vi "Program Deinitialization.vi"(8 "error in":errorcluster, 11 "classes in":T1) -> (0 "error out":errorcluster, 3 "classes out":T1)   [LabVIEW 2011]
uses:
  Controls/Class Objects.ctl
  Modules/File/Configuration/Configuration.lvclass
  Modules/Hardware/Power Supply/Power Supply.lvclass
  Modules/Hardware/Mass Flow Controller/Mass Flow Controller.lvclass
  Modules/Hardware/PID/PID.lvclass
  Modules/Hardware/Valve Controller/Valve Controller.lvclass
  Modules/Hardware/Multimeter/Multimeter.lvclass
  Modules/Hardware/Vapour Generator/Vapour Generator.lvclass
  Modules/File/TDMS/TDMS.lvclass
  Controls/Class Labels.ctl
  Functional Global Data/Globals.ctl
  Functional Global Data/Device Params Global.ctl
  Controls/User Interface Action.ctl
  Controls/Display Mode.ctl
  Functional Global Data/Analysis Data.ctl
  Functional Global Data/Run Data.ctl
  Modules/Menu/Menu Action.ctl
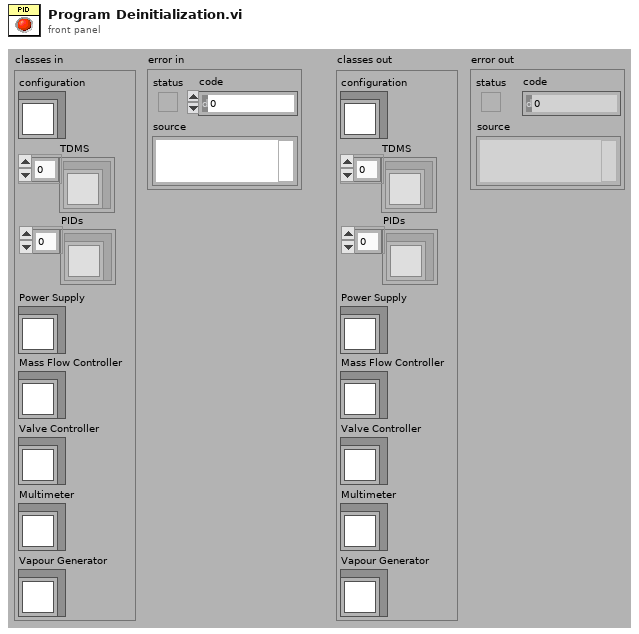
[diagram p1: front panel]
types:
  T1 = typedef "Class Objects.ctl" = cluster{"configuration":refnum<class "Configuration.lvclass">, "TDMS":refnum<class "TDMS.lvclass">[], "Power Supply":refnum<class "Power Supply.lvclass">, "Mass Flow Controller":refnum<class "Mass Flow Controller.lvclass">, "Valve Controller":refnum<class "Valve Controller.lvclass">, "Multimeter":refnum<class "Multimeter.lvclass">, "Vapour Generator":refnum<class "Vapour Generator.lvclass">, "PIDs":refnum<class "PID.lvclass">[]}
  T2 = typedef "Class Labels.ctl" = enum16{"Configuration", "TDMS", "PID", "Power Supply", "Vapour Generator", "MFC", "NMR", "Valve Controller", "Multimeter"}
  T3 = typedef "Globals.ctl" = enum16{"Initialize", "Get DAQ Params", "Get Data Display Params", "Set DAQ Params", "Set Data Display Params"}
  T4 = typedef "Device Params Global.ctl" = enum16{"Initialize", "Get Device Settings", "Get Device Connections", "Set Device Settings", "Set Device Connections", "Get All Device Properties"}
  T5 = typedef "User Interface Action.ctl" = enum16{"Initialize", "Data Acquisition Disable", "Data View Disable", "Sample Set", "Sample Set 2D Data", "Sample Set x0 & dx", "Sample Add", "Sample Set Cursor", "Sample Set Offset & Multiplier", "Sample Set Axis Labels", "Sample Parameters Disabled", "Sample Parameters Update", "Run Update", "Run Set Offset & Multiplier", "Run Set Axis Labels", "Run Set Cursor", "Run Set Disabled", "Run Parameters Update", "Run Parameters Disabled", "Run Number Set", "Run Number Set Range", "Run Number Set Disabled", "Sample Number Set", "Sample Number Set Range", "Notes Set Value", "Update Plot", "Set Plot Parameters", "Update Concentration Plot", "Time Set", "Clear DAQ Display", "Clear Analysis Display", "Status Bar Set", "Progress Bar Set", "Display Mode Set", "Experiment Type Set", "Analysis Plot Average Set", "Stop"}
  T6 = typedef "Display Mode.ctl" = enum16{"Sample", "Run"}
  T7 = typedef "Analysis Data.ctl" = enum16{"Initialize", "Add Plot", "Get Plots"}
  T8 = typedef "Run Data.ctl" = enum16{"Initialize", "Add Sample Channel", "Set Run", "Get Number of Runs", "Set Run Params", "Get Spectrum", "Get Run Params", "Get Sample Params", "Get History", "Get Averaged History", "Get Run Param Names", "Set Run Param Names", "Get Sample Param Names", "Set Sample Param Names", "Get MFC Flow Rate Challenge Profile", "Get History Average"}
  T9 = typedef "Menu Action.ctl" = enum16{"Initialize", "Insert Item", "Remove Item", "Set Checked Item", "Get Checked Item", "Get Item Index", "Item Present?", "Stop"}
  T10 = typedef "Device Connections.ctl" = cluster{"Detector":cluster{"Detector Type":T11, "Connection":bool, "B-M PID":T12, "INL PID Connections":T13}, "Power Supply":cluster{"Type":enum16{"Stanford Research PS350", "Keithley 2400"}, "Connection":bool, "VISA resource name":refnum<visa-resource-name>}, "Mass Flow Controller":cluster{"Type":enum16{"Aalborg GFC17"}, "Connection":bool, "Aalborg GFC17":T15}, "Valve Controller":cluster{"Type":T16, "Connection":bool, "SMC - INL":cluster{"VISA resource name":refnum<visa-resource-name>}}, "Multimeter":cluster{"Multimeter Type":T17, "Connection":bool, "VISA resource name":refnum<visa-resource-name>}, "Vapour Generator":cluster{"Type":T18, "Connection":bool, "Owlstone Gen-SYS":T19}}
  T11 = typedef "Detector Type.ctl" = enum16{"INL PID", "Baseline-Mocon piD-TECH plus"}
  T12 = typedef "Baseline Mocon piD-Tech plus.lvclass/Connections.ctl" = cluster{"AI DAQmx channel":tag}
  T13 = typedef "INL PID Connections.ctl" = cluster{"PIDs":u8, "Integrator DAQ Channels 1":T14, "Integrator DAQ Channels 2":T14}
  T14 = typedef "INL PID.lvclass/Integrator DAQmx Channels.ctl" = cluster{"V0":tag, "S1":tag, "S2":tag}
  T15 = typedef "Aalborg GFC17.lvclass/Aalborg GFC17 Connections.ctl" = cluster{"flow rate setpoint channel":tag, "flow rate reading channel":tag, "valve channel":tag}
  T16 = typedef "Valve Type.ctl" = enum16{"SMC - INL"}
  T17 = typedef "Multimeter Type.ctl" = enum16{"Agilent 3458A"}
  T18 = typedef "Vapour Generator Type.ctl" = enum16{"Owlstone GEN-SYS"}
  T19 = typedef "Owlstone GEN-SYS.lvclass/GEN-SYS Connections.ctl" = cluster{"GEN-SYS VISA resource name":refnum<visa-resource-name>, "OVG-4":cluster{"Flow Address":u8, "Temp Address":u8}, "OHG-4":cluster{"Flow Address":u8, "Easydew VISA resource name":refnum<visa-resource-name>}}
  T20 = typedef "Device Settings.ctl" = cluster{"PID":cluster{"B-M PID":T21, "INL PID":T22}, "Power Supply":cluster{"Source Value":dbl, "Source Value Units":T23, "Source Mode":T24, "Limits":T25, "Output":bool}, "Mass Flow Controller":cluster{"MFC Flow Rate":dbl, "MFC Valve Status":T28}, "Valve Controller":cluster{"Valve Assembly":T29}, "Multimeter":cluster{"Agilent 3458A":cluster{"Measurement Configuration":T31, "Measurement Integration":T32}}, "Vapour Generator":cluster{"Owlstone Permeation Tube":T33, "Owlstone GEN-SYS Setpoints":T35}}
  T21 = typedef "Baseline Mocon piD-Tech plus.lvclass/Settings.ctl" = cluster{"Detector Sampling Frequency":dbl}
  T22 = typedef "INL PID.lvclass/Settings.ctl" = cluster{"Sampling Frequency":dbl, "Integration Time":dbl, "Integration Periods":u8, "Grid Voltage":dbl}
  T23 = typedef "Power Supply.lvclass/Source Units.ctl" = enum16{"volts", "millivolts", "microvolts", "amps", "milliamps", "microamps", "nanoamps"}
  T24 = typedef "Power Supply.lvclass/Source Mode.ctl" = enum16{"Volts", "Current"}
  T25 = typedef "Power Supply.lvclass/Protection Limits.ctl" = cluster{"Voltage Limit":dbl, "Voltage Limit Units":T26, "Current Limit":dbl, "Current Limit Units":T27, "Voltage Trip/Cmpl":dbl, "Voltage Trip/Cmpl Units":T26, "Current Trip/Cmpl":dbl, "Current Trip/Cmpl Units":T27}
  T26 = typedef "Power Supply.lvclass/Voltage Units.ctl" = enum16{"volts", "millivolts", "microvolts"}
  T27 = typedef "Power Supply.lvclass/Current Units.ctl" = enum16{"amps", "milliamps", "microamps", "nanoamps"}
  T28 = typedef "Mass Flow Controller.lvclass/Valve Status.ctl" = enum16{"Open", "Closed"}
  T29 = typedef "Valve Controller.lvclass/Valve Assembly.ctl" = cluster{"Valve 1":T30, "Valve 2":T30, "Valve 3":T30, "Valve 4":T30, "Valve 5":T30}
  T30 = typedef "Valve Controller.lvclass/Status.ctl" = u16
  T31 = typedef "Agilent 3458A.lvclass/Measurement Configuration.ctl" = cluster{"Function":enum16{"DC Voltage", "AC Voltage", "AC + DC Voltage", "DC Current", "AC Current", "AC + DC Current", "2-Wire Resistance", "4-Wire Resistance", "Frequency", "Period", "Direct Sampling DC", "Direct Sampling AC", "Sub-Sampling DC", "Sub-Sampling AC"}, " Manual Resolution":enum16{"4.5", "5.5", "6.5", "7.5", "8.5"}, "Frequency Source":enum16{"AC + DC Current", "AC + DC Voltage", "AC Current", "AC Voltage"}, "Auto Range":enum16{"OFF", "ON", "ONCE"}}
  T32 = typedef "Agilent 3458A.lvclass/Measurement Integration.ctl" = cluster{"Power Line Cycles":dbl}
  T33 = typedef "Owlstone GEN-SYS.lvclass/Permeation Tube.ctl" = cluster{"Tube":T34, "Molecular Weight":dbl, "Calibration Temperature\n(Celcius)":i32, "Permeation Rate \n(ng/min)":i32}
  T34 = typedef "Owlstone GEN-SYS.lvclass/Permeation Tube Gas.ctl" = enum16{"Isobutylene 27 Nov 2012", "Ammonia 29 Sep 2012", "DMMP Tube A 3 July 2014", "DMMP Tube B 3 July 2014"}
  T35 = typedef "Owlstone GEN-SYS.lvclass/Gen-Sys Setpoints.ctl" = cluster{"OVG-4":cluster{"Oven Temperature":i32, "Sample Flow Rate":i32, "Split Flow Status":u16, "Split Flow Rate":i32}, "OHG-4":cluster{"Wet Air Flow":i32}}
  T36 = typedef "Data Acquisition Parameters.ctl" = cluster{"Experiment Type":T37, "Experiment Name":string, "Operator Name":string, "Notes":string, "TDMS File Path":path, "Data Acquisition State":bool, "PID Voltage Sweep":T38, "MFC Challenge Profile - Heaviside Step":T39, "MFC Challenge Profile":T40, "MFC Challenge Profile - Staircase":T41}
  T37 = typedef "DAQ Type.ctl" = enum16{"PID Sample", "PID with PS Challenge", "PID with MFC Challenge", "Multimeter Sample", "Multimeter with MFC Challenge"}
  T38 = typedef "PID Voltage Seep Settings.ctl" = cluster{"Voltage Step (V)":dbl, "Voltage Range (V)":cluster{u16, u16}, "Time Step (s)":dbl, "Voltage Step Direction":enum16{"High 2 Low", "Low 2 High"}}
  T39 = typedef "MFC Challenge Profile - Heaviside Step.ctl" = cluster{"Valve Open Duration":u16, "MFC Flow Rate":dbl, "Valve Open Repeats":u16, "Valve Open Start":u16}
  T40 = typedef "MFC Challen Profile Type.ctl" = enum16{"Heaviside", "Staircase"}
  T41 = typedef "MFC Challenge Profile - Staircase.ctl" = cluster{"Step Time Duration":u16, "Step Flow Rate":dbl, "Steps":u16, "Valve Open Start":u16, "Recovery":bool, "Repeats":u16}
  T42 = enum8{"Enabled", "Disabled", "Disabled and Grayed Out"}
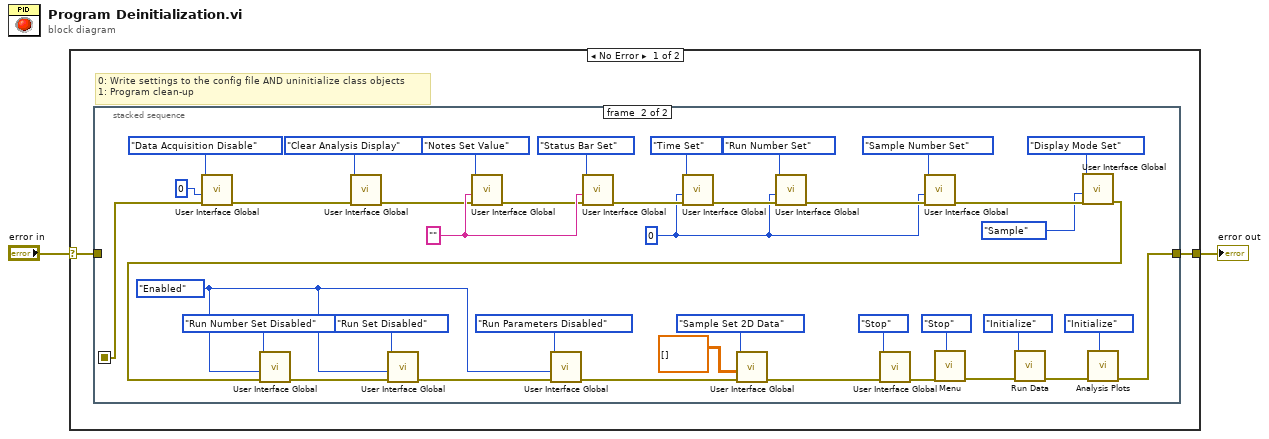
[diagram p0: block diagram]
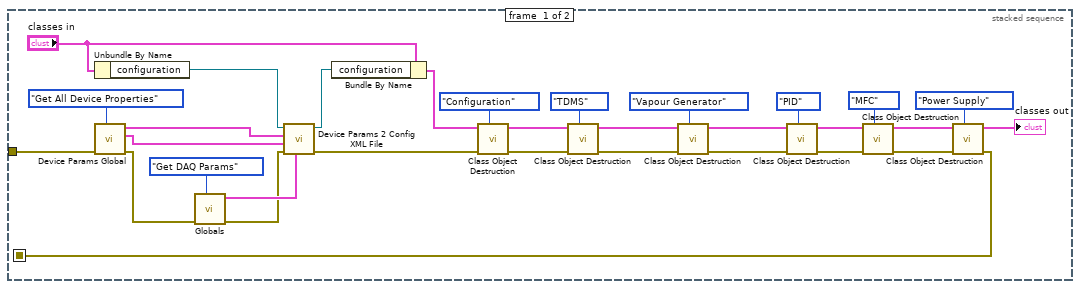
[diagram p2: hidden frame]
diagram:
  n1 = case shown="No Error" "error in" {
    selector: "error in" -> [w3 w75]
    tunnel: [w4 w75] -> w1
    frame No Error {
      # "0: Write settings to the config file AND uninitialize class objects\n1: Program clean-up"
      n2 = stacked-sequence {
        seq-local: [w5 _] -> [_ w64]
        tunnel: [_ w63] -> w4
        tunnel: w3 -> [w15 _]
        frame #0 {
          n3 = Unbundle By Name("classes in") -> ("configuration"=w35:refnum<class "Configuration.lvclass">)
          n4 = call "Device Params Global.vi"("action"=Device_Params_Global."Get All Device Properties", "error in"=w15) -> ("error out"=w11:errorcluster, "Device Connections OUT"=w13:T10, "Device Settings OUT"=w17:T20)  [unwired: 7 in]
          n5 = call "Globals.vi"("action"=Globals."Get DAQ Params", "error in"=w11) -> ("error out"=w12:errorcluster, "Data Acquisition"=w14:T36)  [unwired: 7 in, 1 out]
          n6 = call "Device Params 2 Config XML File.vi"("Data Acquisition Parameters"=w14, "error in"=w12, "Device Connections"=w13, "Device Settings"=w17, "Configuration in"=w35) -> ("error out"=w20:errorcluster, "Configuration out"=w33:refnum<class "Configuration.lvclass">)  [unwired: 4 in]
          n7 = Bundle By Name(cluster="classes in", "configuration"=w33) -> (w19:T1)
          n8 = call "Class Object Destruction.vi"("class labels"=Class_Labels."Configuration", "error in"=w20, "classes in"=w19) -> ("error out"=w23:errorcluster, "classes out"=w24:T1)  [unwired: 7 in]
          n9 = call "Class Object Destruction.vi"("class labels"=Class_Labels."TDMS", "error in"=w23, "classes in"=w24) -> ("error out"=w9:errorcluster, "classes out"=w7:T1)  [unwired: 7 in]
          n10 = call "Class Object Destruction.vi"("class labels"=Class_Labels."Vapour Generator", "error in"=w9, "classes in"=w7) -> ("error out"=w8:errorcluster, "classes out"=w6:T1)  [unwired: 7 in]
          n11 = call "Class Object Destruction.vi"("class labels"=Class_Labels."PID", "error in"=w8, "classes in"=w6) -> ("error out"=w28:errorcluster, "classes out"=w27:T1)  [unwired: 7 in]
          n12 = call "Class Object Destruction.vi"("class labels"=Class_Labels."MFC", "error in"=w28, "classes in"=w27) -> ("error out"=w30:errorcluster, "classes out"=w31:T1)  [unwired: 7 in]
          n13 = call "Class Object Destruction.vi"("class labels"=Class_Labels."Power Supply", "error in"=w30, "classes in"=w31) -> ("error out"=w5:errorcluster, "classes out"=→"classes out":T1)  [unwired: 7 in]
        }
        frame #1 {
          w40 = T42."Enabled" ("Disabled")
          w51 = 0 ("Time (s)")
          w59 = ""
          n14 = call "User Interface Global.vi"("error in"=w64, "data1"=0, "action"=User_Interface_Action."Data Acquisition Disable" ("Action")) -> ("error out"=w69:errorcluster)  [unwired: 8 in]
          n15 = call "User Interface Global.vi"("error in"=w69, "action"=User_Interface_Action."Clear Analysis Display") -> ("error out"=w50:errorcluster)  [unwired: 9 in]
          n16 = call "User Interface Global.vi"("error in"=w50, "data1"=w59, "action"=User_Interface_Action."Notes Set Value") -> ("error out"=w58:errorcluster)  [unwired: 8 in]
          n17 = call "User Interface Global.vi"("error in"=w58, "data1"=w59, "action"=User_Interface_Action."Status Bar Set") -> ("error out"=w56:errorcluster)  [unwired: 8 in]
          n18 = call "User Interface Global.vi"("error in"=w56, "data1"=w51, "action"=User_Interface_Action."Time Set") -> ("error out"=w54:errorcluster)  [unwired: 8 in]
          n19 = call "User Interface Global.vi"("error in"=w54, "data1"=w51, "action"=User_Interface_Action."Run Number Set") -> ("error out"=w52:errorcluster)  [unwired: 8 in]
          n20 = call "User Interface Global.vi"("error in"=w52, "data1"=w51, "action"=User_Interface_Action."Sample Number Set") -> ("error out"=w45:errorcluster)  [unwired: 8 in]
          n21 = call "User Interface Global.vi"("error in"=w45, "data1"=Display_Mode."Sample" ("Display Mode"), "action"=User_Interface_Action."Display Mode Set") -> ("error out"=w39:errorcluster)  [unwired: 8 in]
          n22 = call "User Interface Global.vi"("error in"=w39, "data1"=w40, "action"=User_Interface_Action."Run Number Set Disabled") -> ("error out"=w38:errorcluster)  [unwired: 8 in]
          n23 = call "User Interface Global.vi"("error in"=w38, "data1"=w40, "action"=User_Interface_Action."Run Set Disabled") -> ("error out"=w37:errorcluster)  [unwired: 8 in]
          n24 = call "User Interface Global.vi"("error in"=w37, "data1"=w40, "action"=User_Interface_Action."Run Parameters Disabled") -> ("error out"=w36:errorcluster)  [unwired: 8 in]
          n25 = call "User Interface Global.vi"("error in"=w36, "data1"=dbl[][] [], "action"=User_Interface_Action."Sample Set 2D Data") -> ("error out"=w47:errorcluster)  [unwired: 8 in]
          n26 = call "User Interface Global.vi"("error in"=w47, "action"=User_Interface_Action."Stop" ("Action")) -> ("error out"=w72:errorcluster)  [unwired: 9 in]
          n27 = call "Menu.vi"("action"=Menu_Action."Stop" ("Menu"), "error in"=w72) -> ("error out"=w68:errorcluster)  [unwired: 6 in, 3 out]
          n28 = call "Run Data.vi"("error in"=w68, "action"=Run_Data."Initialize" ("Action")) -> ("error out"=w67:errorcluster)  [unwired: 6 in, 3 out]
          n29 = call "Analysis Plots.vi"("action"=Analysis_Data."Initialize" ("Action"), "error in"=w67) -> ("error out"=w63:errorcluster)  [unwired: 7 in, 2 out]
        }
      }
    }
    frame Error {
    }
  }
  "error out" <- w1
